vi "获取配置文件.vi"(8 "错误输入":errorcluster) -> (0 "错误输出":errorcluster, 1 "路径输出":path, 3 "数组":string[](array[string]))   [LabVIEW 2021]
panel:
  out "文件名":string[](array[string])
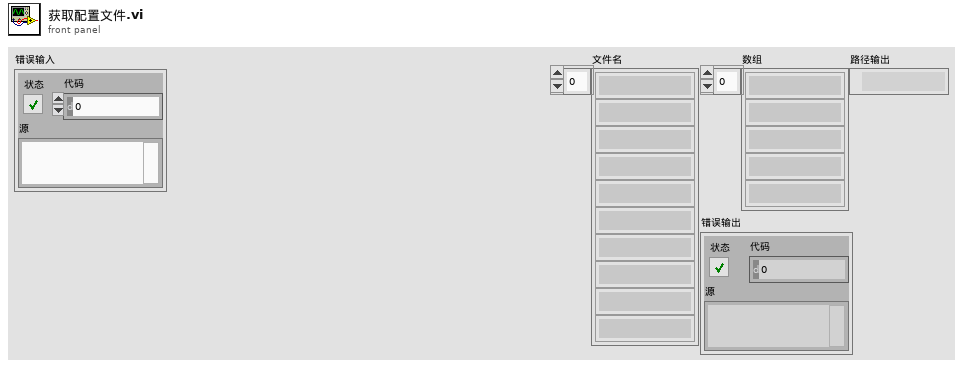
[diagram p1: front panel]
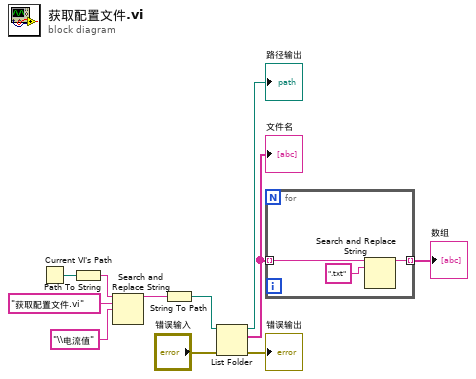
[diagram p0: block diagram]
diagram:
  n1 = Current VI's Path() -> (path=w6:path)
  n2 = Path To String(path=w6) -> (string=w2:string)
  n3 = Search and Replace String(input string=w2, search string="获取配置文件.vi" ("搜索字符串"), replace string="\\电流值" ("字符串")) -> (result string=w3:string)  [unwired: 5 in, 3 out]
  n4 = String To Path(string=w3) -> (path=w5:path)
  n5 = List Folder(path=w5, error in="错误输入") -> (path out=→"路径输出":path, filenames=w11:string[], error out=→"错误输出":errorcluster)  [unwired: 2 in, 1 out]
  "文件名" <- w11
  n6 = for {
    tunnel: w11 -> [w14] mode=indexing
    tunnel: [w12] -> w10 mode=indexing
    n7 = Search and Replace String(input string=w14, search string=".txt" ("搜索字符串")) -> (result string=w12:string)  [unwired: 6 in, 3 out]
  }
  "数组" <- w10
